vi "Readable String.vi"(11 "SeqRunning Condition in":refnum<class "SeqRunning Condition.lvclass">) -> (2 "String":string)   [LabVIEW 2020, in "VolatusSeq.lvlib" / "SeqRunning Condition.lvclass"]
uses:
  SeqRunning Condition.lvclass
  SeqRunning Condition.lvclass/SeqRunning Condition.ctl
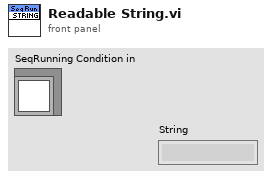
[diagram p1: front panel]
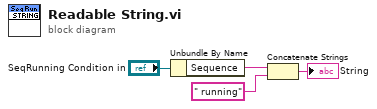
[diagram p0: block diagram]
diagram:
  n1 = Unbundle By Name("SeqRunning Condition in") -> ("Sequence"=w4:string)
  n2 = Concatenate Strings(w4, " running" ("string")) -> (→"String":string)
